vi "GlobalReg.vi"() -> ()   [LabVIEW 2013]
panel:
  in  "SimulatedAO0":i16
  out "DMAsOverflow15":bool
  out "DMAsOverflow14":bool
  out "DMAsOverflow13":bool
  out "DMAsOverflow12":bool
  out "DMAsOverflow11":bool
  out "DMAsOverflow10":bool
  out "DMAsOverflow9":bool
  out "DMAsOverflow8":bool
  out "DMAsOverflow7":bool
  out "DMAsOverflow6":bool
  out "DMAsOverflow5":bool
  out "DMAsOverflow4":bool
  out "DMAsOverflow3":bool
  out "DMAsOverflow2":bool
  out "DMAsOverflow1":bool
  out "DMAsOverflow0":bool
  out "DMAsOverflow":u16
  in  "GroupEnable5":bool
  in  "SamplingRate5":u16=10000
  in  "GroupEnable4":bool
  in  "SamplingRate4":u16=10000
  in  "GroupEnable3":bool
  in  "SamplingRate3":u16=10000
  in  "GroupEnable2":bool
  in  "SamplingRate2":u16=10000
  in  "GroupEnable1":bool
  in  "SamplingRate1":u16=10000
  in  "GroupEnable0":bool
  in  "SamplingRate0":u16=10000
  in  "DebugMode":bool
  in  "DAQStartStop":bool
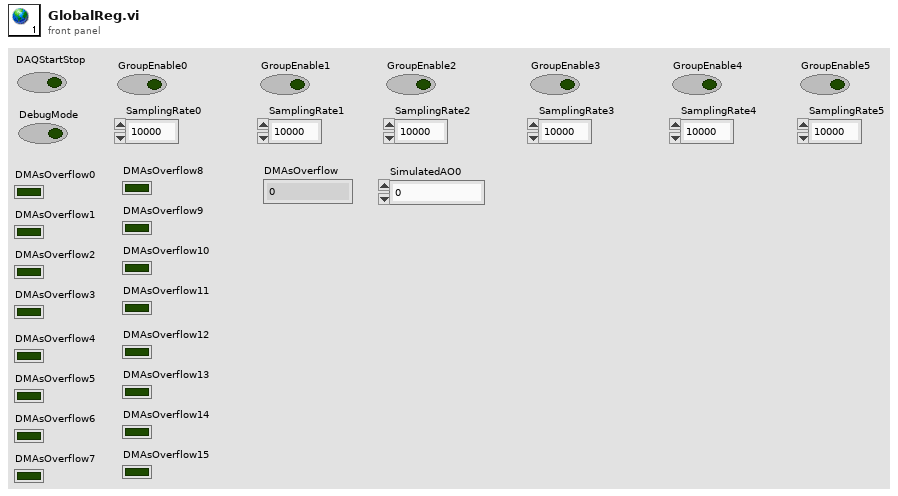
[diagram p1: front panel]
diagram:
